vi "Create Resources.vi"(0 "channel":u8) -> (4 "channel collection builder":refnum<class "Collection Builder.lvclass">, 15 "channel":refnum<class "niUSRP Channel v1 FPGA.lvclass">)   [LabVIEW 2023, in "niUSRP Channel v1 FPGA.lvclass"]
uses:
  <instrlib>/niVST/Reference FPGA/FPGA/Channel/niUSRP Channel v1 FPGA.lvclass
  <instrlib>/niVST/Reference FPGA/FPGA/Channel/Regs.ctl
  <vilib>/rvi/LocalResourceManager/LocalResourceManager.xnode
  <vilib>/rvi/DataTransferAndStorage/Container/Common/niFpgaContainerGetUniqueNameForEmu.vi
  <vilib>/rvi/DataTransferAndStorage/Container/Common/niFpgaContainerSetEmuInfo.vi
  <vilib>/rvi/eio/common/nirviEmuReportErrorAndStop.vi
  <instrlib>/_niInstr/Instruction Framework/v1/FPGA/Collection Builder/Collection Builder.lvclass
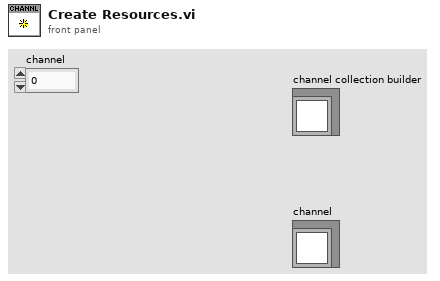
[diagram p1: front panel]
types:
  T1 = typedef "niUSRP Channel v1 FPGA.lvclass/Regs.ctl" = cluster{"enable":refnum<k21>, "reset":refnum<k21>, "channel no.":u8}
  T2 = typedef "niInstr Address Space Collection Builder v1 FPGA.lvlib/Parent Metadata.ctl" = cluster{"UID":u16, "version":u16, "oldest compatible version":u16}
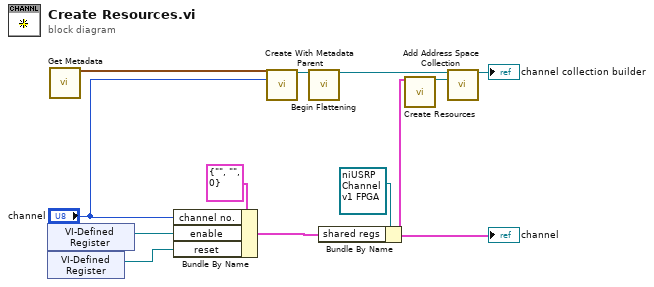
[diagram p0: block diagram]
diagram:
  n1 = xnode "VI-Defined Register"() -> ("Register Out"=w10:refnum<k21>)
  n2 = xnode "VI-Defined Register"() -> ("Register Out"=w9:refnum<k21>)
  n3 = call <instrlib>:"Get Metadata.vi"() -> ("shared metadata"=w7:T2)  [unwired: 15 in]
  n4 = Bundle By Name(cluster=T1 {"enable"="", "reset"="", "channel no."=0} ("rx regs"), "channel no."="channel", "enable"=w10, "reset"=w9) -> (w2:T1)
  n5 = call <instrlib>:"Create With Metadata Parent.vi"("parent metadata"=w7, "instance (0)"="channel") -> ("collection builder"=w6:refnum<class "Collection Builder.lvclass">)  [unwired: 13 in]
  n6 = call <instrlib>:"Begin Flattening.vi"("collection builder in"=w6) -> ("collection builder out"=w5:refnum<class "Collection Builder.lvclass">)  [unwired: 14 in]
  n7 = Bundle By Name(cluster=refnum<class "niUSRP Channel v1 FPGA.lvclass"> refnum, "shared regs"=w2) -> (w3:cluster{})
  "channel" <- w3
  n8 = call <instrlib>:"Create Resources.vi"("address space"=w3) -> ("single address space collection"=w4:refnum<class "Single Address Space Collection.lvclass">)  [unwired: 14 in]
  n9 = call <instrlib>:"Add Address Space Collection.vi"("collection builder in"=w5, "address space collection"=w4) -> ("collection builder out"=→"channel collection builder":refnum<class "Collection Builder.lvclass">)  [unwired: 13 in]
